vi "release queues.vi"(0 "display queues":T1, 7 "disk queues":T1, 11 "error in (no error)":errorcluster) -> (15 "error out":errorcluster)   [LabVIEW 2017]
uses:
  typedefs/queue cluster.ctl
  typedefs/reading queue.ctl
  typedefs/reading.ctl
  typedefs/readingType.ctl
  typedefs/reading 1 queue.ctl
  typedefs/reading1.ctl
  popup panels/control panel globals.vi
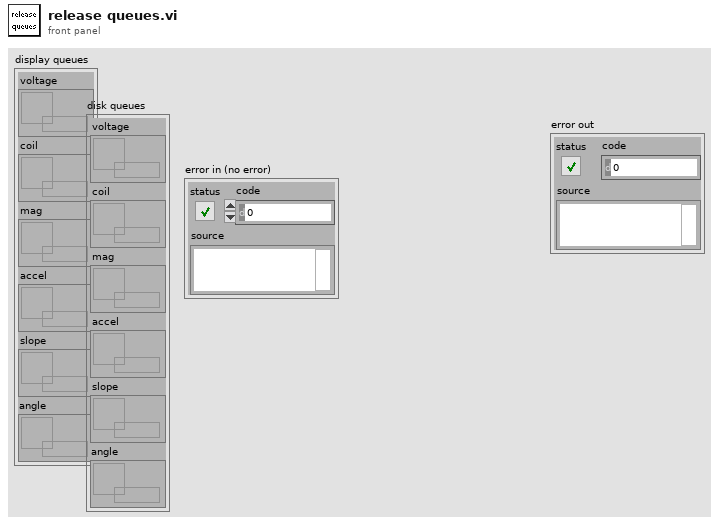
[diagram p1: front panel]
types:
  T1 = typedef "queue cluster.ctl" = cluster{"voltage":T2, "coil":T2, "mag":T2, "accel":T2, "slope":T3, "angle":T2}
  T2 = typedef "reading queue.ctl" = refnum<queue>
  T3 = typedef "reading 1 queue.ctl" = refnum<queue>
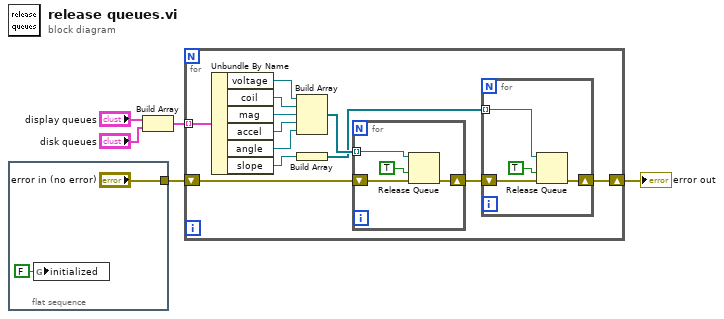
[diagram p0: block diagram]
diagram:
  n1 = flat-sequence {
    tunnel: ["error in (no error)"] -> w2
    frame #0 {
      n2 = global write "control panel globals.vi" "initialized"(FALSE ("initialized")) -> ()
    }
  }
  n3 = Build Array("display queues", "disk queues") -> (w3:T1[])
  n4 = for {
    tunnel: w3 -> [w19] mode=indexing
    shift-right: [w9] -> w1
    shift-left: w2 -> [w12]
    n5 = Unbundle By Name(w19) -> ("voltage"=w18:T2, "coil"=w17:T2, "mag"=w16:T2, "accel"=w15:T2, "angle"=w8:T2, "slope"=w14:T3)
    n6 = Build Array(w18, w17, w16, w15, w8) -> (w13:T2[])
    n7 = Build Array(w14) -> (w11:T3[])
    n8 = for {
      tunnel: w13 -> [w27] mode=indexing
      shift-right: [w25] -> w10
      shift-left: w12 -> [w24]
      n9 = Release Queue(queue=w27, force destroy? (F)=TRUE, error in (no error)=w24) -> (error out=w25:errorcluster)  [unwired: 2 out]
    }
    n10 = for {
      tunnel: w11 -> [w23] mode=indexing
      shift-right: [w21] -> w9
      shift-left: w10 -> [w20]
      n11 = Release Queue(queue=w23, force destroy? (F)=TRUE, error in (no error)=w20) -> (error out=w21:errorcluster)  [unwired: 2 out]
    }
  }
  "error out" <- w1
